vi "Contour Line_Find Intersected Edges (col).vi"(6 "|/|? (F)":bool, 7 "col":i32, 8 "height":dbl, 9 "Z":dbl[][](array[numeric]), 10 "Y":dbl[][](array[numeric]), 11 "X":dbl[][](array[numeric])) -> (2 "Intersected Edges":T1(array[cluster]), 3 "Contour Points":cluster{"x":dbl, "y":dbl}[](array[cluster]))   [LabVIEW 2017, in "NI_AAL_Geometry.lvlib"]
uses:
  <vilib>/Analysis/NI_AAL_Geometry.lvlib
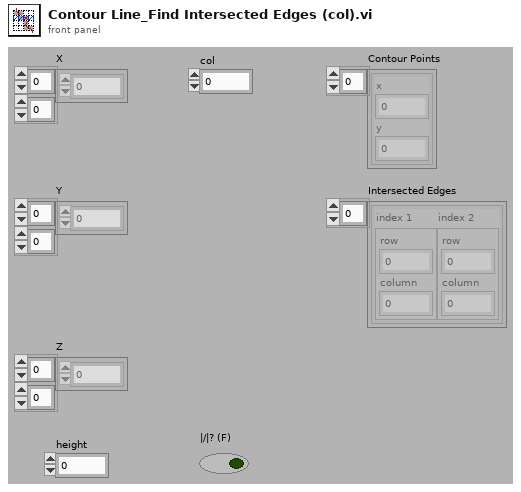
[diagram p1: front panel]
types:
  T1 = cluster{"index 1":cluster{"row":i32, "column":i32}, "index 2":cluster{"row":i32, "column":i32}}[]
  T2 = cluster{"index 1":cluster{"row":i32, "column":i32}, "index 2":cluster{"row":i32, "column":i32}}
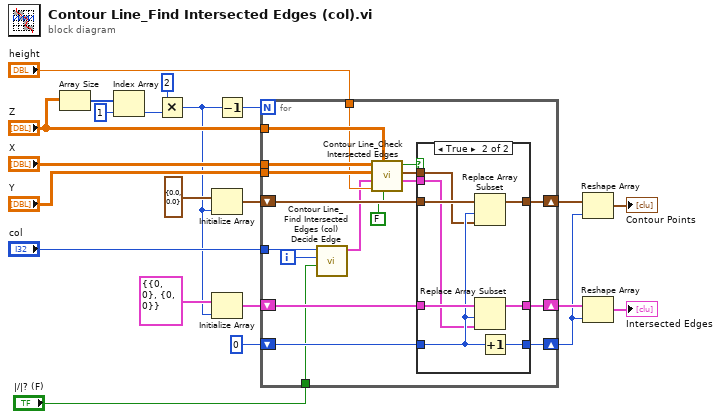
[diagram p0: block diagram]
diagram:
  n1 = Array Size(array="Z") -> (size(s)=w22:i32[])
  n2 = Index Array(array=w22, index=1) -> (element=w4:i32)
  n3 = Multiply(x=2, y=w4) -> (x*y=w6:i32)
  n4 = Initialize Array(cluster{"x":dbl, "y":dbl} {"x"=0.0, "y"=0.0} ("contour point"), w6) -> (w18:cluster{"x":dbl, "y":dbl}[])
  n5 = Initialize Array(T2 {"index 1"={"row"=0, "column"=0}, "index 2"={"row"=0, "column"=0}} ("intersected edge"), w6) -> (w17:T1)
  n6 = Decrement(x=w6) -> (x-1=w9:i32)
  n7 = for {
    N: w9 -> [_]
    tunnel: "col" -> [w27]
    tunnel: "height" -> [w29]
    tunnel: "X" -> [w34]
    tunnel: "Y" -> [w33]
    shift-right: [w39] -> w3
    shift-left: w18 -> [w40]
    shift-right: [w37] -> w2
    shift-left: w17 -> [w38]
    shift-right: [w35] -> w1
    shift-left: 0 -> [w36]
    tunnel: "|/|? (F)" -> [w24]
    tunnel: "Z" -> [w32]
    i -> [w25]
    n8 = call <vilib>:"Contour Line_Find Intersected Edges (col) Decide Edge.vi"("|/|? (F)"=w24, "index"=w25, "col"=w27) -> ("edge"=w26:T2)  [unwired: 8 out]
    n9 = call <vilib>:"Contour Line_Check Intersected Edges.vi"("row? (F)"=FALSE, "Z"=w32, "height"=w29, "edge in"=w26, "Y"=w33, "X"=w34) -> ("edge out"=w30:T2, "contour point"=w31:cluster{"x":dbl, "y":dbl}, "intersected?"=w28:bool)  [unwired: 3 out]
    n10 = case shown="True" w28 {
      tunnel: w40 -> [w43 w51]
      tunnel: [w43 w50] -> w39
      tunnel: w38 -> [w42 w49]
      tunnel: [w42 w48] -> w37
      tunnel: w36 -> [w41 w47]
      tunnel: [w41 w46] -> w35
      tunnel: w31 -> [_ w45]
      tunnel: w30 -> [_ w44]
      frame False {
      }
      frame True {
        n11 = Replace Array Subset(array=w51, new element=w45, index=w47) -> (w50:cluster{"x":dbl, "y":dbl}[])
        n12 = Replace Array Subset(array=w49, new element=w44, index=w47) -> (w48:T1)
        n13 = Increment(x=w47) -> (x+1=w46:i32)
      }
    }
  }
  n14 = Reshape Array(w3, w1) -> (→"Contour Points":cluster{"x":dbl, "y":dbl}[])
  n15 = Reshape Array(w2, w1) -> (→"Intersected Edges":T1)
